vi "PIM Limit Key Array.vi"(4 "Conversion":enum16{"Cluster - HTML", "HTML - Cluster"}(ring), 6 "PIM Test Parameters":T1={"Stimulus"={"C1 Pwr dBm"=0.0, "C2 Pwr dBm"=0.0, "Power Units"=enum."dBm", "Meas Type"=enum."Time", "C1 Freq MHz"=0.0, "C2 Freq MHz"=0.0, "Swept Freq Step"=0}, "Measure"={"IM Order"=0, "Direction"=0, "Averaging"=1, "ALC ON?"=TRUE, "Peak Hold?"=TRUE, "Peak last N"=1, "Ref Level dBm"=-100.0, "Ref Units"=enum."dBm", "Num Samples"=1, "Sample units"=enum."Sample(s)", "Update Rate (s)"=0.0, "DUT PORT"=enum."Port 1", "Percent (%)"=100}, "Display"={"Power Scale"={"yRange_min"=0, "yRange_max"=0}, "xRange_span"=5}} {"Stimulus"."Swept Freq Step" items=[".2", ".4", "1.0", "2.0"]; "Measure"."Averaging" items=["None", "Minimum", "Normal", "High", "Maximum"]; "Measure"."Direction" items=["Reverse", "Forward", "Auxiliary"]; "Measure"."IM Order" items=["3rd", "5th", "7th", "9th", "11th", "13th", "15th", "17th", "19th", "21st", "23rd", "25th", "27th", "29th", "31st", "33rd"]}, 7 "Key Array In":T11) -> (1 "PIM Test Parameters (out)":T1={"Stimulus"={"C1 Pwr dBm"=0.0, "C2 Pwr dBm"=0.0, "Power Units"=enum."dBm", "Meas Type"=enum."Time", "C1 Freq MHz"=0.0, "C2 Freq MHz"=0.0, "Swept Freq Step"=0}, "Measure"={"IM Order"=0, "Direction"=0, "Averaging"=1, "ALC ON?"=TRUE, "Peak Hold?"=TRUE, "Peak last N"=1, "Ref Level dBm"=-100.0, "Ref Units"=enum."dBm", "Num Samples"=1, "Sample units"=enum."Sample(s)", "Update Rate (s)"=0.0, "DUT PORT"=enum."Port 1", "Percent (%)"=100}, "Display"={"Power Scale"={"yRange_min"=0, "yRange_max"=0}, "xRange_span"=5}} {"Stimulus"."Swept Freq Step" items=[".2", ".4", "1.0", "2.0"]; "Measure"."Averaging" items=["None", "Minimum", "Normal", "High", "Maximum"]; "Measure"."Direction" items=["Reverse", "Forward", "Auxiliary"]; "Measure"."IM Order" items=["3rd", "5th", "7th", "9th", "11th", "13th", "15th", "17th", "19th", "21st", "23rd", "25th", "27th", "29th", "31st", "33rd"]}, 2 "Key Array Out":T11)   [LabVIEW 2011]
uses:
  ITK/utils/keyedarr.llb/Keyed Array.ctl
  TypeDefs/PIM Test Parameters.ctl
  TypeDefs/PIM Stimulus Parameters.ctl
  BPIMCore/HW IO/PIM Sweep Step Size.ctl
  TypeDefs/PIM Measurement Parameters.ctl
  BPIMCore/HW IO/IMOrder.ctl
  BPIMCore/HW IO/MeasMode.ctl
  BPIMCore/HW IO/HW Averaging.ctl
  TypeDefs/PIM Meas Units.ctl
  BPIMCore/HW IO/DUTport.ctl
  TypeDefs/PIM Display Parameters.ctl
  ITK/utils/strutil.llb/Case Matching.ctl
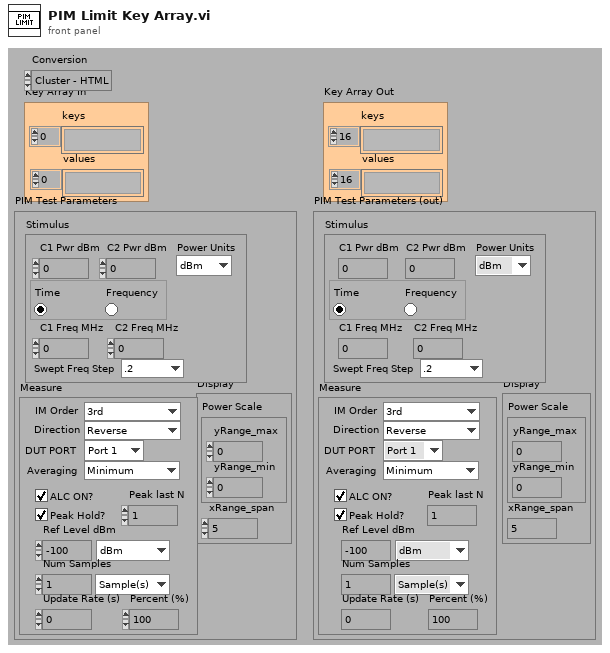
[diagram p1: front panel]
types:
  T1 = typedef "PIM Test Parameters.ctl" = cluster{"Stimulus":T2, "Measure":T4, "Display":T10}
  T2 = typedef "PIM Stimulus Parameters.ctl" = cluster{"C1 Pwr dBm":dbl, "C2 Pwr dBm":dbl, "Power Units":enum16{"dBm", "Watts"}, "Meas Type":enum32{"Time", "Frequency"}, "C1 Freq MHz":dbl, "C2 Freq MHz":dbl, "Swept Freq Step":T3}
  T3 = typedef "PIM Sweep Step Size.ctl" = u16
  T4 = typedef "PIM Measurement Parameters.ctl" = cluster{"IM Order":T5, "Direction":T6, "Averaging":T7, "ALC ON?":bool, "Peak Hold?":bool, "Peak last N":u32, "Ref Level dBm":dbl, "Ref Units":enum16{"dBm", "dBc"}, "Num Samples":u32, "Sample units":T8, "Update Rate (s)":dbl, "DUT PORT":T9, "Percent (%)":u8}
  T5 = typedef "IMOrder.ctl" = u8
  T6 = typedef "MeasMode.ctl" = u16
  T7 = typedef "HW Averaging.ctl" = u16
  T8 = typedef "PIM Meas Units.ctl" = enum16{"Sample(s)", "Second(s)", "Sweep(s)"}
  T9 = typedef "DUTport.ctl" = enum16{"Port 1", "Port 2"}
  T10 = typedef "PIM Display Parameters.ctl" = cluster{"Power Scale":cluster{"yRange_min":i32, "yRange_max":i32}, "xRange_span":u32}
  T11 = typedef "Keyed Array.ctl" = cluster{"keys":string[], "values":string[]}
  T12 = typedef "Case Matching.ctl" = enum16{"a != A", "a == A", "system"}
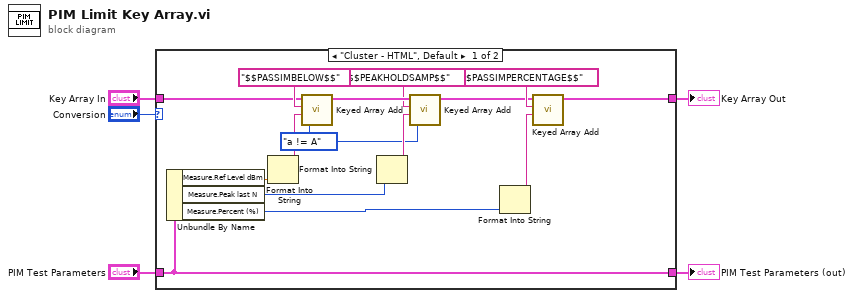
[diagram p0: block diagram]
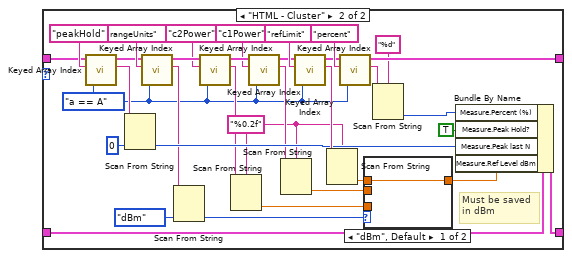
[diagram p2: hidden frame]
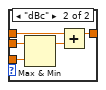
[diagram p3: hidden frame]
diagram:
  n1 = case shown="\"Cluster - HTML\", Default" "Conversion" {
    tunnel: "Key Array In" -> [w17 w47]
    tunnel: "PIM Test Parameters" -> [w12 w54]
    tunnel: [w6 w25] -> w3
    tunnel: [w12 w53] -> w2
    frame "Cluster - HTML", Default {
      w11 = Case_Matching."a != A" ("case matching (sensitive)")
      n2 = Unbundle By Name(w12) -> ("Measure.Ref Level dBm"=w16:dbl, "Measure.Peak last N"=w14:u32, "Measure.Percent (%)"=w9:u8)
      n3 = Format Into String(w16) -> (resulting string=w15:string)  [unwired: 3 in, 1 out]
      n4 = call "Keyed Array Add.vi"("case matching (sensitive)"=w11, "value"=w15, "key"="$$PASSIMBELOW$$", "array in"=w17) -> ("array out"=w20:T11)  [unwired: 3 out]
      n5 = Format Into String(w14) -> (resulting string=w13:string)  [unwired: 3 in, 1 out]
      n6 = call "Keyed Array Add.vi"("case matching (sensitive)"=w11, "value"=w13, "key"="$$PEAKHOLDSAMP$$", "array in"=w20) -> ("array out"=w7:T11)  [unwired: 3 out]
      n7 = Format Into String(w9) -> (resulting string=w8:string)  [unwired: 3 in, 1 out]
      n8 = call "Keyed Array Add.vi"("value"=w8, "key"="$$PASSIMPERCENTAGE$$", "array in"=w7) -> ("array out"=w6:T11)  [unwired: 1 in, 3 out]
    }
    frame "HTML - Cluster" {
      w29 = "%0.2f" ("format string")
      w24 = Case_Matching."a == A" ("case matching (sensitive)")
      # "Must be saved\nin dBm"
      n9 = call "Keyed Array Index.vi"("case matching (sensitive)"=w24, "key"="peakHold", "array in"=w47) -> ("value"=w49:string, "duplicate array"=w41:T11)  [unwired: 1 in, 2 out]
      n10 = Scan From String(input string=w49, default 1=0 ("Display.Power Scale.yRange_min")) -> (output 1=w45:i32)  [unwired: 3 in, 3 out]
      n11 = call "Keyed Array Index.vi"("case matching (sensitive)"=w24, "key"="rangeUnits", "array in"=w41) -> ("value"=w43:string, "duplicate array"=w36:T11)  [unwired: 1 in, 2 out]
      n12 = Scan From String(input string=w43, default 1=enum16{"dBm", "dBc"}."dBm" ("Measure.Ref Units")) -> (output 1=w33:enum16{"dBm", "dBc"})  [unwired: 3 in, 3 out]
      n13 = call "Keyed Array Index.vi"("case matching (sensitive)"=w24, "key"="c2Power", "array in"=w36) -> ("value"=w39:string, "duplicate array"=w40:T11)  [unwired: 1 in, 2 out]
      n14 = Scan From String(format string=w29, input string=w39) -> (output 1=w31:dbl)  [unwired: 2 in, 4 out]
      n15 = call "Keyed Array Index.vi"("case matching (sensitive)"=w24, "key"="c1Power", "array in"=w40) -> ("value"=w38:string, "duplicate array"=w35:T11)  [unwired: 1 in, 2 out]
      n16 = Scan From String(format string=w29, input string=w38) -> (output 1=w32:dbl)  [unwired: 2 in, 4 out]
      n17 = call "Keyed Array Index.vi"("case matching (sensitive)"=w24, "key"="refLimit", "array in"=w35) -> ("value"=w52:string, "duplicate array"=w26:T11)  [unwired: 1 in, 2 out]
      n18 = Scan From String(format string=w29, input string=w52) -> (output 1=w30:dbl)  [unwired: 2 in, 4 out]
      n19 = call "Keyed Array Index.vi"("case matching (sensitive)"=w24, "key"="percent", "array in"=w26) -> ("value"=w23:string, "duplicate array"=w25:T11)  [unwired: 1 in, 2 out]
      n20 = case shown="\"dBm\", Default" w33 {
        tunnel: w32 -> [_ w60]
        tunnel: w31 -> [_ w59]
        tunnel: w30 -> [w55 w57]
        tunnel: [w55 w56] -> w28
        frame "dBm", Default {
        }
        frame "dBc" {
          n21 = Max & Min(x=w60, y=w59) -> (max(x,y)=w58:dbl)  [unwired: 1 out]
          n22 = Add(x=w57, y=w58) -> (x+y=w56:dbl)
        }
      }
      n23 = Scan From String(format string="%d", input string=w23) -> (output 1=w22:i32)  [unwired: 2 in, 4 out]
      n24 = Bundle By Name(cluster=w54, "Measure.Percent (%)"=w22, "Measure.Peak Hold?"=TRUE, "Measure.Peak last N"=w45, "Measure.Ref Level dBm"=w28) -> (w53:T1)
    }
  }
  "Key Array Out" <- w3
  "PIM Test Parameters (out)" <- w2
